vi "Main.vi"(8 "error in (no error)":errorcluster, 11 "Plugin Thread in":refnum<class "Plugin Thread.lvclass">) -> (0 "error out":errorcluster, 3 "Plugin Thread out":refnum<class "Plugin Thread.lvclass">)   [LabVIEW 2017, in "DSF Core.lvlib" / "Plugin Thread.lvclass"]
uses:
  Thread/Plugin/Plugin Thread.lvclass
  Thread/Plugin/Plugin Thread.lvclass/Plugin Thread.ctl
  Interfaces/Interface/Interface.lvclass/Interface.ctl
  Transfer Group/Transfer Group.lvclass/Transfer Group.ctl
  Timing/Timing.lvclass/Timing.ctl
  Interfaces/Transceiver Interface/Read.vi
  Interfaces/Transceiver Interface/Read Plugin Command.vi
  Get Interface.vi
  Transfer Group/Write Return FIFO.vi
  Interfaces/Interface/Read Command.vi
  Transfer Group/Get Return FIFO.vi
  Transfer Group/Get Timing.vi
  Timing/Get Iteration.vi
  Interfaces/Interface/Read RT FIFO(16B).vi
  Interfaces/Transceiver Interface/Plugin Interface.lvclass
  C:/Git/DSF/Data Sharing Framework/Source/Core/Engine/Classes/Interfaces/Interface/Interface.lvclass
  Interfaces/Interface/Errors.vi
  Interfaces/Interface/Command Timeout.vi
  Thread Pool/Return Plugin Interface.vi
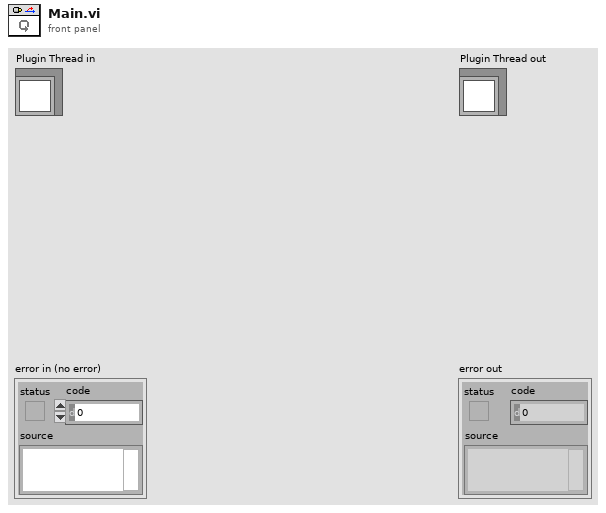
[diagram p1: front panel]
types:
  T1 = typedef "DSF Core.lvlib/Plugin Interface.lvclass/Command Data.ctl" = cluster{"Command":T2, "Command Parameters":T3}
  T2 = typedef "DSF Core.lvlib/Plugin Interface.lvclass/Command.ctl" = enum8{"Set Inline Buffer", "Rx", "Tx", "Shutdown"}
  T3 = typedef "DSF Core.lvlib/Plugin Interface.lvclass/Command Parameters.ctl" = cluster{"arg1":u64, "arg2":u64}
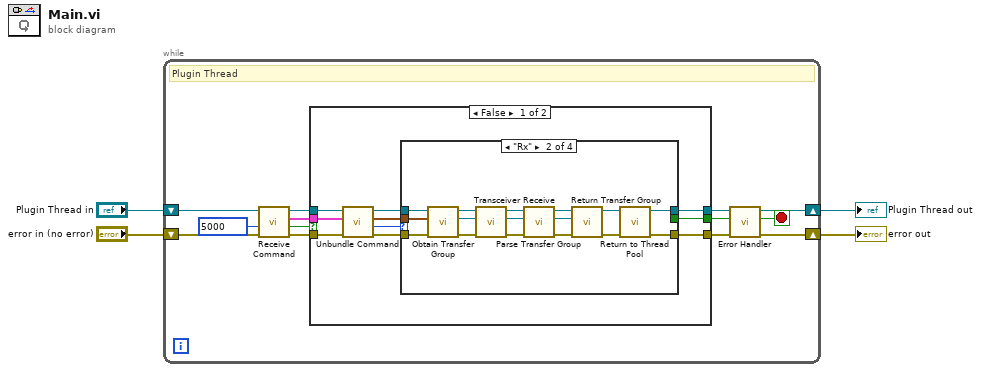
[diagram p0: block diagram]
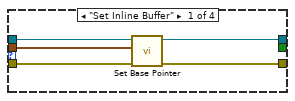
[diagram p2: hidden frame]
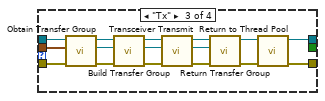
[diagram p3: hidden frame]
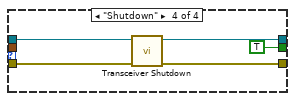
[diagram p4: hidden frame]
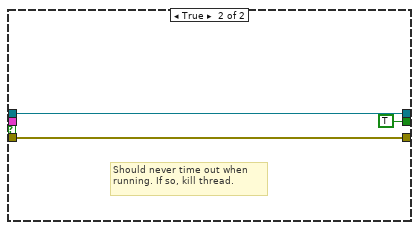
[diagram p5: hidden frame]
diagram:
  n1 = while {
    shift-right: [w12] -> w1
    shift-left: "error in (no error)" -> [w17]
    shift-right: [w13] -> w2
    shift-left: "Plugin Thread in" -> [w16]
    stop <- w11 stop-if-true
    # "Plugin Thread"
    n2 = call "Receive Command.vi"("error in (no error)"=w17, "timeout in ms (0)"=5000 ("timeout in ms"), "Plugin Thread in"=w16) -> ("error out"=w5:errorcluster, "timed out?"=w6:bool, "command"=w7:T1, "Plugin Thread out"=w8:refnum<class "Plugin Thread.lvclass">)  [unwired: 5 in]
    n3 = case shown="False" w6 {
      tunnel: w8 -> [w25 w72]
      tunnel: [w27 w72] -> w15
      tunnel: w5 -> [w24 w71]
      tunnel: w7 -> [w23 _]
      tunnel: [w26 w71] -> w14
      tunnel: [w18 TRUE] -> w10
      frame False {
        n4 = call "Unbundle Command.vi"("error in (no error)"=w24, "command"=w23, "Plugin Thread in"=w25) -> ("error out"=w21:errorcluster, "command"=w22:T2, "command parameters"=w19:T3, "Plugin Thread out"=w20:refnum<class "Plugin Thread.lvclass">)  [unwired: 5 in]
        n5 = case shown="\"Rx\"" w22 {
          tunnel: w20 -> [w32 w38 w54 w69]
          tunnel: [w31 w40 w57 w67] -> w27
          tunnel: w21 -> [w28 w33 w53 w68]
          tunnel: w19 -> [w29 w37 w50 _]
          tunnel: [w30 w39 w56 w66] -> w26
          tunnel: [_ _ _ TRUE] -> w18
          frame "Set Inline Buffer" {
            n6 = call "Set Base Pointer.vi"("error in (no error)"=w28, "command parameters"=w29, "Plugin Thread in"=w32) -> ("error out"=w30:errorcluster, "Plugin Thread out"=w31:refnum<class "Plugin Thread.lvclass">)  [unwired: 7 in]
          }
          frame "Rx" {
            n7 = call "Obtain Transfer Group.vi"("error in (no error)"=w33, "command parameters"=w37, "Transceiver Thread in"=w38) -> ("error out"=w35:errorcluster, "Transfer Group"=w34:refnum<class "Transfer Group.lvclass">, "Transceiver Thread out"=w36:refnum<class "Plugin Thread.lvclass">)  [unwired: 6 in]
            n8 = call "Transceiver Receive.vi"("error in (no error)"=w35, "Transfer Group in"=w34, "Transceiver Thread in"=w36) -> ("error out"=w47:errorcluster, "Transfer Group out"=w46:refnum<class "Transfer Group.lvclass">, "Transceiver Thread out"=w48:refnum<class "Plugin Thread.lvclass">)  [unwired: 6 in]
            n9 = call "Parse Transfer Group.vi"("error in (no error)"=w47, "Transfer Group in"=w46, "Plugin Thread in"=w48) -> ("error out"=w44:errorcluster, "Transfer Group out"=w43:refnum<class "Transfer Group.lvclass">, "Plugin Thread out"=w45:refnum<class "Plugin Thread.lvclass">)  [unwired: 6 in]
            n10 = call "Return Transfer Group.vi"("error in (no error)"=w44, "Transfer Group"=w43, "Transceiver Thread in"=w45) -> ("error out"=w41:errorcluster, "Transceiver Thread out"=w42:refnum<class "Plugin Thread.lvclass">)  [unwired: 7 in]
            n11 = call "Return to Thread Pool.vi"("error in (no error)"=w41, "Plugin Thread in"=w42) -> ("error out"=w39:errorcluster, "Plugin Thread out"=w40:refnum<class "Plugin Thread.lvclass">)  [unwired: 8 in]
          }
          frame "Tx" {
            n12 = call "Obtain Transfer Group.vi"("error in (no error)"=w53, "command parameters"=w50, "Transceiver Thread in"=w54) -> ("error out"=w51:errorcluster, "Transfer Group"=w49:refnum<class "Transfer Group.lvclass">, "Transceiver Thread out"=w52:refnum<class "Plugin Thread.lvclass">)  [unwired: 6 in]
            n13 = call "Build Transfer Group.vi"("error in (no error)"=w51, "Transfer Group in"=w49, "Plugin Thread in"=w52) -> ("error out"=w63:errorcluster, "Transfer Group out"=w55:refnum<class "Transfer Group.lvclass">, "Plugin Thread out"=w64:refnum<class "Plugin Thread.lvclass">)  [unwired: 6 in]
            n14 = call "Transceiver Transmit.vi"("error in (no error)"=w63, "Transfer Group in"=w55, "Transceiver Thread in"=w64) -> ("error out"=w61:errorcluster, "Transfer Group out"=w60:refnum<class "Transfer Group.lvclass">, "Transceiver Thread out"=w62:refnum<class "Plugin Thread.lvclass">)  [unwired: 6 in]
            n15 = call "Return Transfer Group.vi"("error in (no error)"=w61, "Transfer Group"=w60, "Transceiver Thread in"=w62) -> ("error out"=w58:errorcluster, "Transceiver Thread out"=w59:refnum<class "Plugin Thread.lvclass">)  [unwired: 7 in]
            n16 = call "Return to Thread Pool.vi"("error in (no error)"=w58, "Plugin Thread in"=w59) -> ("error out"=w56:errorcluster, "Plugin Thread out"=w57:refnum<class "Plugin Thread.lvclass">)  [unwired: 8 in]
          }
          frame "Shutdown" {
            n17 = call "Transceiver Shutdown.vi"("error in (no error)"=w68, "Transceiver Thread in"=w69) -> ("error out"=w66:errorcluster, "Transceiver Thread out"=w67:refnum<class "Plugin Thread.lvclass">)  [unwired: 8 in]
          }
        }
      }
      frame True {
        # "Should never time out when running. If so, kill thread."
      }
    }
    n18 = call "Error Handler.vi"("error in (no error)"=w14, "stop"=w10, "Plugin Thread in"=w15) -> ("error out"=w12:errorcluster, "stop"=w11:bool, "Plugin Thread out"=w13:refnum<class "Plugin Thread.lvclass">)  [unwired: 6 in]
  }
  "error out" <- w1
  "Plugin Thread out" <- w2
